vi "Select Channels.vi"(8 "error in (no error)":errorcluster, 9 "Channel":string[](array[string]), 10 "Table Name":string, 11 "[V]System Tree View in":refnum<class "[V]System Tree View.lvclass">) -> (0 "error out":errorcluster, 3 "[V]System Tree View out":refnum<class "[V]System Tree View.lvclass">)   [LabVIEW 2020, in "[V]System Tree View.lvlib" / "[V]System Tree View.lvclass"]
uses:
  [V]System Tree View.lvclass
  [V]System Tree View.lvclass/[V]System Tree View.ctl
  Depden On/MVVM Framework/MVVM Abstruct View/MVVM Abstruct View/MVVM Abstruct View.lvclass/MVVM Abstruct View.ctl
  Models/Data Loader/Data Load Interface/Data Load Interface Messages/Select Channel Msg/Select Channel Msg.lvclass/Select Channel Msg.ctl
  <vilib>/ActorFramework/Message Enqueuer/Message Enqueuer.lvclass/Message Enqueuer.ctl
  7d85db43-8c9e-43de-a6b4-b91cfa38546d.vi
  Depden On/MVVM Framework/MVVM Abstruct View/MVVM Abstruct View/Accessor/Read ActorMap-Models.vi
  7d85db43-8c9e-43de-a6b4-b91cfa38546d.vi/d4db2432-cc9c-482c-8957-dac855435ef6.vi
  7d85db43-8c9e-43de-a6b4-b91cfa38546d.vi/86fbf154-bd7b-49a2-8ab2-a837b2a95f24.vi
  7d85db43-8c9e-43de-a6b4-b91cfa38546d.vi/3b95b01e-1ec2-4565-bcd9-7606a5281010.vi
  7d85db43-8c9e-43de-a6b4-b91cfa38546d.vi/96a08935-737a-44b2-979c-a81d56408f7e.vi
  <vilib>/ActorFramework/Message Enqueuer/Enqueue.vi
  7d85db43-8c9e-43de-a6b4-b91cfa38546d.vi/d4db2432-cc9c-482c-8957-dac855435ef6.vi/6eaecd13-6e48-4772-a921-b51ebdf84d88.vi
  7d85db43-8c9e-43de-a6b4-b91cfa38546d.vi/d4db2432-cc9c-482c-8957-dac855435ef6.vi/d2d5f2b7-06f4-47f6-971c-049c3fdbb653.vi
  7d85db43-8c9e-43de-a6b4-b91cfa38546d.vi/3b95b01e-1ec2-4565-bcd9-7606a5281010.vi/6eaecd13-6e48-4772-a921-b51ebdf84d88.vi
  7d85db43-8c9e-43de-a6b4-b91cfa38546d.vi/3b95b01e-1ec2-4565-bcd9-7606a5281010.vi/d2d5f2b7-06f4-47f6-971c-049c3fdbb653.vi
  7d85db43-8c9e-43de-a6b4-b91cfa38546d.vi/96a08935-737a-44b2-979c-a81d56408f7e.vi/6eaecd13-6e48-4772-a921-b51ebdf84d88.vi
  7d85db43-8c9e-43de-a6b4-b91cfa38546d.vi/96a08935-737a-44b2-979c-a81d56408f7e.vi/d2d5f2b7-06f4-47f6-971c-049c3fdbb653.vi
  Models/Data Loader/Data Load Interface/Data Load Interface Messages/Select Channel Msg/Select Channel Msg.lvclass
  C:/Program Files (x86)/National Instruments/LabVIEW 2020/vi.lib/ActorFramework/Message/Message.lvclass
  <vilib>/ActorFramework/Message Priority Queue/Priority Enqueue.vi
  Depden On/ActorMap/ActorMap.lvclass
  <vilib>/Comparison/Less/Less Functor/Less Functor.lvclass
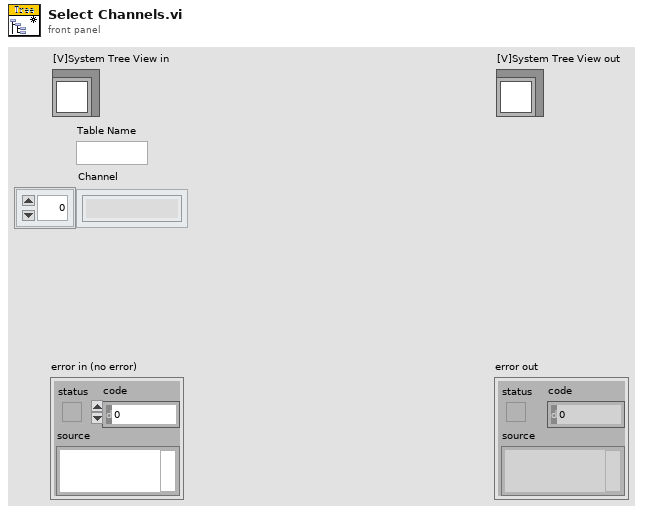
[diagram p1: front panel]
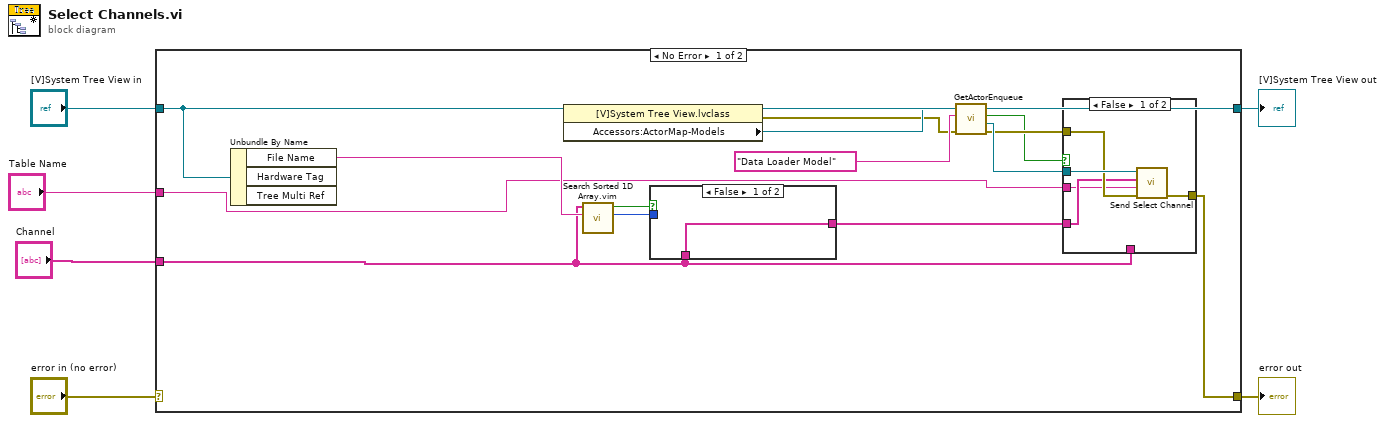
[diagram p0: block diagram]
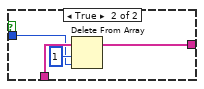
[diagram p2: hidden frame]
diagram:
  n1 = case shown="No Error" "error in (no error)" {
    selector: "error in (no error)" -> [_ w34]
    tunnel: [w14 w34] -> w5
    tunnel: [w20 w33] -> w3
    tunnel: "[V]System Tree View in" -> [w21 w33]
    tunnel: "Channel" -> [w9 _]
    tunnel: "Table Name" -> [w7 _]
    frame No Error {
      n2 = Unbundle By Name(w21) -> ("File Name"=w13:string)  [unwired: 2 out]
      n3 = property class="[V]System Tree View.lvclass"(reference=w21) -> (reference out=w20:refnum<class "[V]System Tree View.lvclass">, error out=w16:errorcluster, "Accessors:ActorMap-Models"=w19:refnum<class "ActorMap.lvclass">)  [unwired: 1 in]
      n4 = call "Search Sorted 1D Array.vim"("element"=w13, "sorted 1D array"=w9) -> ("nearest index"=w10:i32, "found?"=w12:bool)  [unwired: 8 in]
      n5 = case shown="False" w12 {
        tunnel: w10 -> [_ w24]
        tunnel: w9 -> [w22 w26]
        tunnel: [w22 w23] -> w8
        frame False {
        }
        frame True {
          n6 = Delete From Array(array=w26, length=1, index=w24) -> (array with subset deleted=w23:string[])  [unwired: 1 out]
        }
      }
      n7 = call "GetActorEnqueue.vi"("error in (no error)"=w16, "name"="Data Loader Model", "ActorMap in"=w19) -> ("error out"=w15:errorcluster, "Enqueue"=w17:refnum<class "Message Enqueuer.lvclass">, "key not found?"=w11:bool)  [unwired: 5 in, 1 out]
      n8 = case shown="False" w11 {
        tunnel: w17 -> [w31 _]
        tunnel: w15 -> [w30 w32]
        tunnel: [w29 w32] -> w14
        tunnel: w9 -> [_ _]
        tunnel: w8 -> [w28 _]
        tunnel: w7 -> [w27 _]
        frame False {
          n9 = call "Send Select Channel.vi"("error in (no error)"=w30, "Table Name"=w27, "Select Channels"=w28, "Message Enqueuer"=w31) -> ("error out"=w29:errorcluster)  [unwired: 6 in, 1 out]
        }
        frame True {
        }
      }
    }
    frame Error {
    }
  }
  "error out" <- w5
  "[V]System Tree View out" <- w3
